vi "SetStageToScanPixel.vi"(0 "SCAN":bool, 5 "STEP":bool, 7 "Stage Setup Info":T1, 9 "At Point":bool, 11 "error in (no error)":errorcluster) -> (1 "X Pixel":i32, 3 "X (mm)":dbl, 4 "Completed?":bool, 6 "Active":bool, 10 "As Expected?":bool, 12 "Y Pixel":i32, 14 "Y (mm)":dbl, 15 "error out":errorcluster)   [LabVIEW 2018]
uses:
  Controls/StageInfo.ctl
  Program_Files/Labview2018/MAIN/instr.lib/ASI TG-1000/Public/Utility/Axis Name.ctl
  Program_Files/Labview2018/MAIN/instr.lib/_niInstr/Basic Elements/v1/FPGA/niInstr Basic Elements v1 FPGA.lvlib
  Program_Files/Labview2018/MAIN/instr.lib/ASI TG-1000/ASI TG-1000.lvlib
panel:
  out "Positions [internal units]":dbl[](array[numeric])
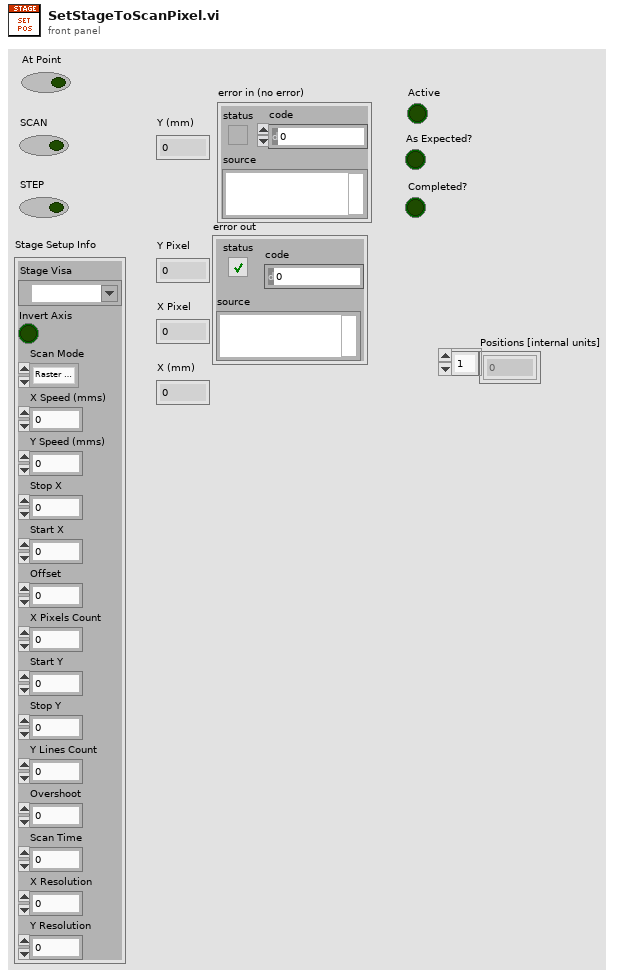
[diagram p1: front panel]
types:
  T1 = typedef "StageInfo.ctl" = cluster{"Stage Visa":refnum<visa-resource-name>, "Invert Axis":bool, "Scan Mode":enum16{"Raster Scan", "Serpentine Scan"}, "X Speed (mms)":dbl, "Y Speed (mms)":dbl, "Stop X":dbl, "Start X":dbl, "Offset":dbl, "X Pixels Count":i32, "Start Y":dbl, "Stop Y":dbl, "Y Lines Count":i32, "Overshoot":dbl, "Scan Time":dbl, "X Resolution":dbl, "Y Resolution":dbl}
  T2 = typedef "ASI TG-1000.lvlib/Axis Name.ctl" = enum8{"undefined", "A", "B", "C", "D", "E", "F", "G", "H", "I", "J", "K", "L", "M", "N", "O", "P", "Q", "R", "S", "T", "U", "V", "W", "X", "Y", "Z"}
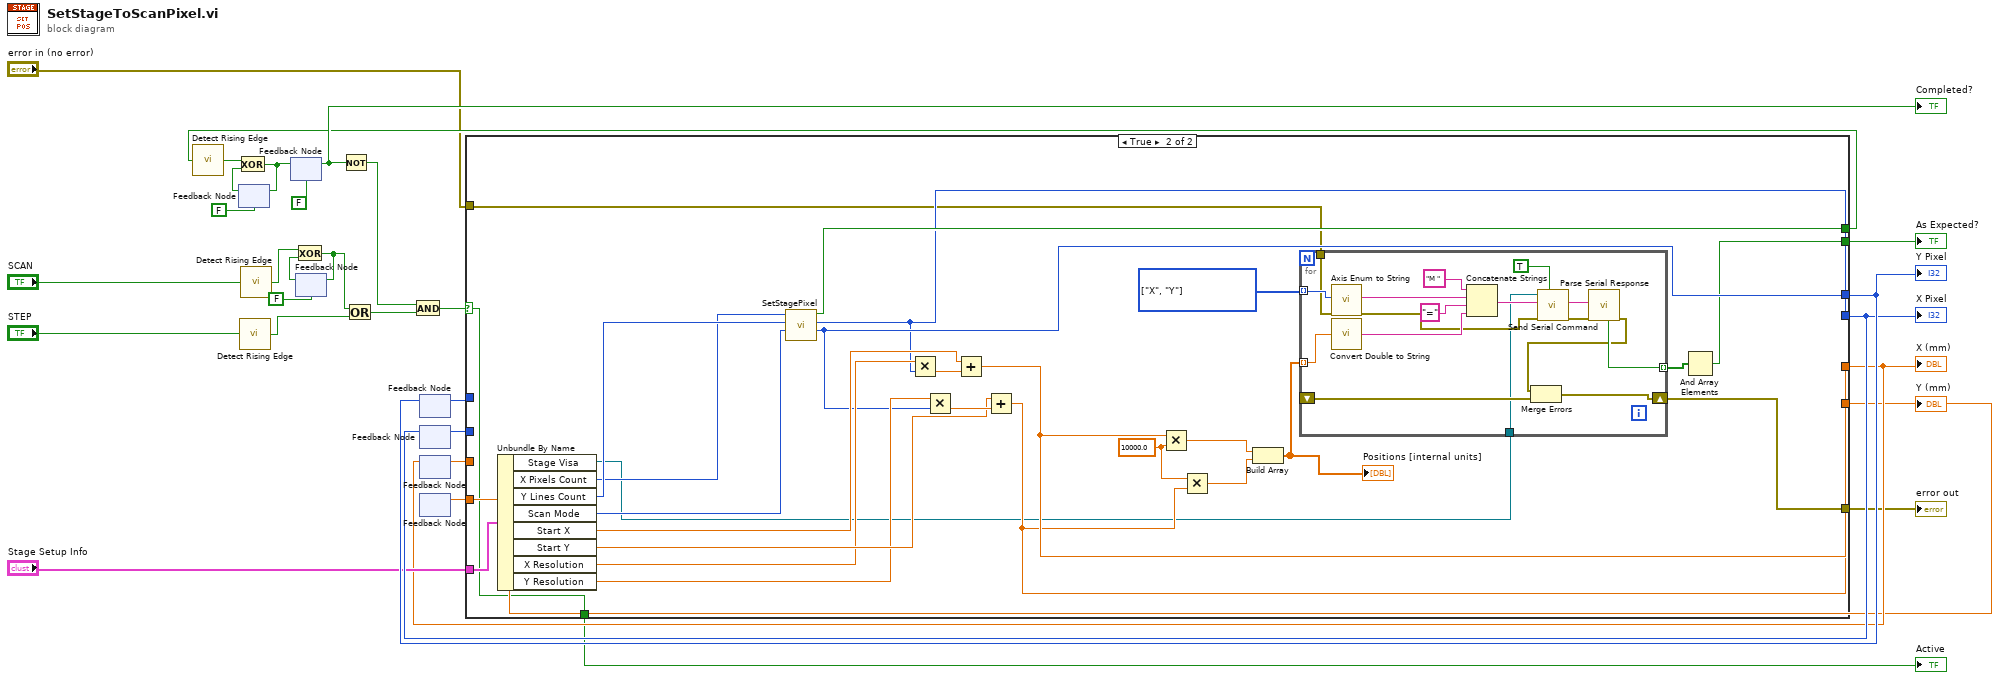
[diagram p0: block diagram]
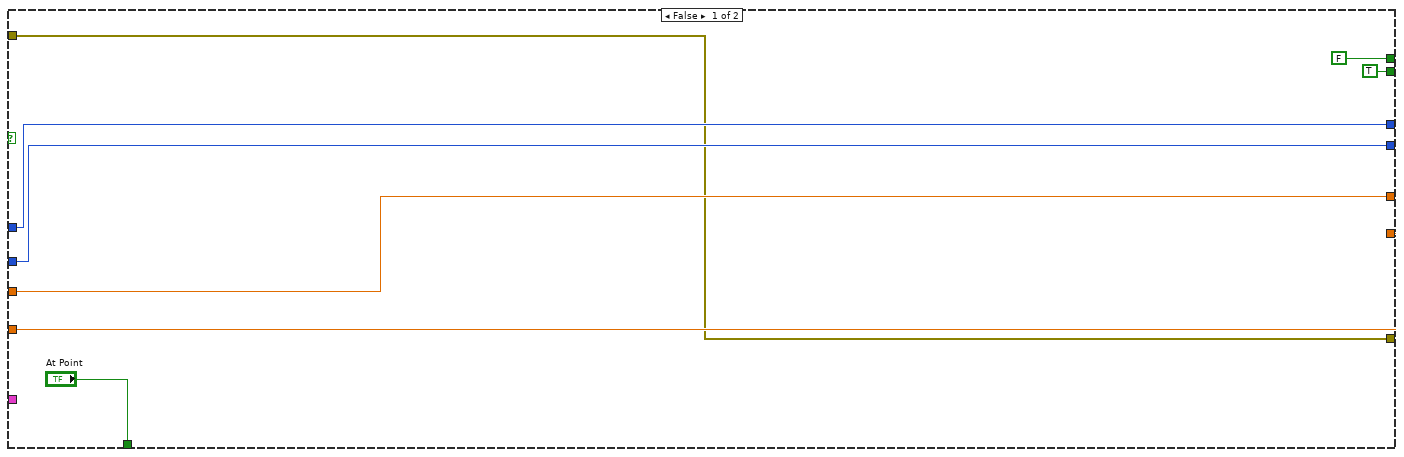
[diagram p2: hidden frame]
diagram:
  n1 = feedback #1(FALSE ("output")) -> (w19:bool)
  n2 = call "Detect Rising Edge.vi"("signal"="STEP") -> ("edge detected"=w9:bool)  [unwired: 14 in]
  n3 = call "Detect Rising Edge.vi"("signal"="SCAN") -> ("edge detected"=w11:bool)  [unwired: 14 in]
  n4 = feedback #2(FALSE ("output")) -> (w24:bool)
  "Completed?" <- w24
  n5 = feedback #3(FALSE ("output")) -> (w14:bool)
  n6 = Exclusive Or(1:w14, 2:w11) -> (0:w13:bool)
  n7 = feedback-in #3(w13) -> ()
  n8 = Not(x=w24) -> (.not. x?=w18:bool)
  n9 = Or(x=w13, y=w9) -> (x .or. y?=w15:bool)
  n10 = And(x=w18, y=w15) -> (x .and. y?=w16:bool)
  n11 = feedback #4() -> (w25:i32)  [unwired: 1 in]
  n12 = feedback #5() -> (w26:i32)  [unwired: 1 in]
  n13 = feedback #6() -> (w27:dbl)  [unwired: 1 in]
  n14 = feedback #7() -> (w28:dbl)  [unwired: 1 in]
  n15 = case shown="True" w16 {
    selector: w16 -> [_ w40]
    tunnel: [FALSE ("Completed?") w64] -> w23
    tunnel: "Stage Setup Info" -> [_ w62]
    tunnel: [w35 w51] -> w6
    tunnel: [w34 w50] -> w5
    tunnel: [w37 w53] -> w30
    tunnel: [w36 w52] -> w29
    tunnel: w25 -> [w37 _]
    tunnel: w26 -> [w36 _]
    tunnel: w27 -> [w35 _]
    tunnel: w28 -> [w34 _]
    tunnel: "error in (no error)" -> [w32 w43]
    tunnel: [w32 w42] -> w4
    tunnel: [TRUE w41] -> w2
    tunnel: ["At Point" w40] -> w1
    frame False {
    }
    frame True {
      w46 = T2[] [enum."X", enum."Y"] items=["undefined", "A", "B", "C", "D", "E", "F", "G", "H", "I", "J", "K", "L", "M", "N", "O", "P", "Q", "R", "S", "T", "U", "V", "W", "X", "Y", "Z"] ("Array of axes")
      w47 = 10000.0 ("x")
      n16 = Unbundle By Name(w62) -> ("Stage Visa"=w39:refnum<visa-resource-name>, "X Pixels Count"=w60:i32, "Y Lines Count"=w61:i32, "Scan Mode"=w63:enum16{"Raster Scan", "Serpentine Scan"}, "Start X"=w57:dbl, "Start Y"=w56:dbl, "X Resolution"=w55:dbl, "Y Resolution"=w54:dbl)
      n17 = call "SetStagePixel.vi"("Scan Mode"=w63, "Line Count"=w61, "Pixel Count"=w60) -> ("Y Pixel"=w53:i32, "X Pixel"=w52:i32, "Completed?"=w64:bool)  [unwired: 6 in]
      n18 = Multiply(x=w55, y=w52) -> (x*y=w59:dbl)
      n19 = Multiply(x=w54, y=w53) -> (x*y=w58:dbl)
      n20 = Add(x=w57, y=w59) -> (x+y=w51:dbl)
      n21 = Add(x=w56, y=w58) -> (x+y=w50:dbl)
      n22 = Multiply(x=w51, y=w47) -> (x*y=w48:dbl)
      n23 = Multiply(x=w47, y=w50) -> (x*y=w49:dbl)
      n24 = Build Array(w48, w49) -> (w45:dbl[])
      "Positions [internal units]" <- w45
      n25 = for {
        tunnel: w46 -> [w73] mode=indexing
        tunnel: w45 -> [w74] mode=indexing
        tunnel: [w71] -> w44 mode=indexing
        shift-right: [w68] -> w42
        shift-left: _ -> [w70]
        tunnel: w43 -> [w66]
        tunnel: w39 -> [w65]
        n26 = call "Axis Enum to String.vi"("error in (no error)"=w66, "Axis Enum In"=w73) -> ("error out"=w72:errorcluster, "Axis String Out"=w78:string)  [unwired: 8 in]
        n27 = call "Convert Double to String.vi"("Value"=w74) -> ("String"=w77:string)
        n28 = Concatenate Strings("M " ("Command"), w78, "=" ("string"), w77) -> (w80:string)
        n29 = call "Send Serial Command.vi"("Listen for response (T)"=TRUE, "error in (no error)"=w72, "Command"=w80, "VISA in"=w65) -> ("error out"=w76:errorcluster, "Response"=w75:string)  [unwired: 5 in, 1 out]
        n30 = call "Parse Serial Response.vi"("error in (no error)"=w76, "Raw Response"=w75) -> ("error out"=w69:errorcluster, "As expected?"=w71:bool)  [unwired: 6 in, 2 out]
        n31 = Merge Errors(w69, w70) -> (w68:errorcluster)
      }
      n32 = And Array Elements(Boolean array=w44) -> (logical AND=w41:bool)
    }
  }
  "Y Pixel" <- w30
  "X Pixel" <- w29
  "Y (mm)" <- w5
  "X (mm)" <- w6
  "error out" <- w4
  "As Expected?" <- w2
  "Active" <- w1
  n33 = call "Detect Rising Edge.vi"("signal"=w23) -> ("edge detected"=w21:bool)  [unwired: 14 in]
  n34 = Exclusive Or(1:w19, 2:w21) -> (0:w22:bool)
  n35 = feedback-in #1(w22) -> ()
  n36 = feedback-in #2(w22) -> ()
  n37 = feedback-in #4(w30) -> ()
  n38 = feedback-in #5(w29) -> ()
  n39 = feedback-in #6(w6) -> ()
  n40 = feedback-in #7(w5) -> ()
